vi "OxITC503 _Config_ Write AUTO-PID table.vi"(3 "error in":errorcluster, 4 "AUTOPID Table in":T1(array[cluster]), 5 "VISA session in":refnum<visa-resource-name>) -> (0 "error out":errorcluster, 1 "AUTOPID Table out":T1(array[cluster]), 2 "VISA session out":refnum<visa-resource-name>)   [LabVIEW 2013]
doc: "NOTE: this VI uses ITC503'specialist commands.\n\nWrites ITC503's AUTO-PID table. The AUTO-PID table is a 32x4 matrix of real numbers. Changes are not permanently stored (use ITC store routine to save PID table within ITC)."
panel:
  in  "Write PID Table to Instrument":bool
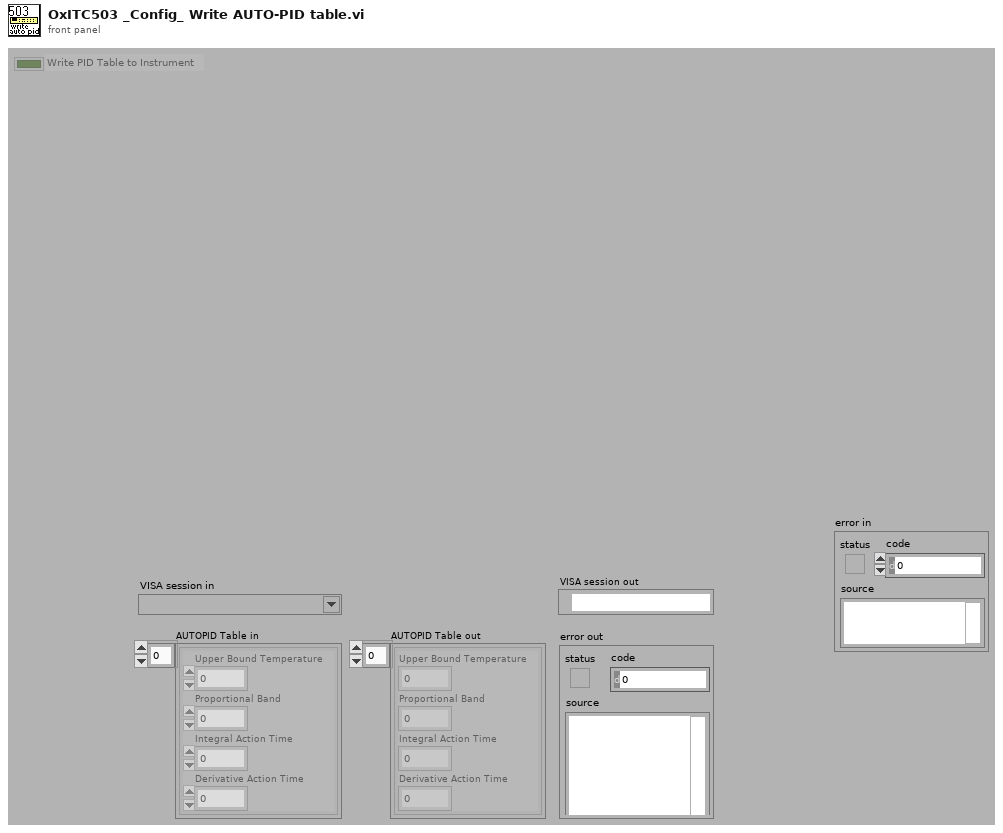
[diagram p1: front panel]
types:
  T1 = cluster{"Upper Bound Temperature":dbl, "Proportional Band":dbl, "Integral Action Time":dbl, "Derivative Action Time":dbl}[]
  T2 = cluster{"Upper Bound Temperature":dbl, "Proportional Band":dbl, "Integral Action Time":dbl, "Derivative Action Time":dbl}
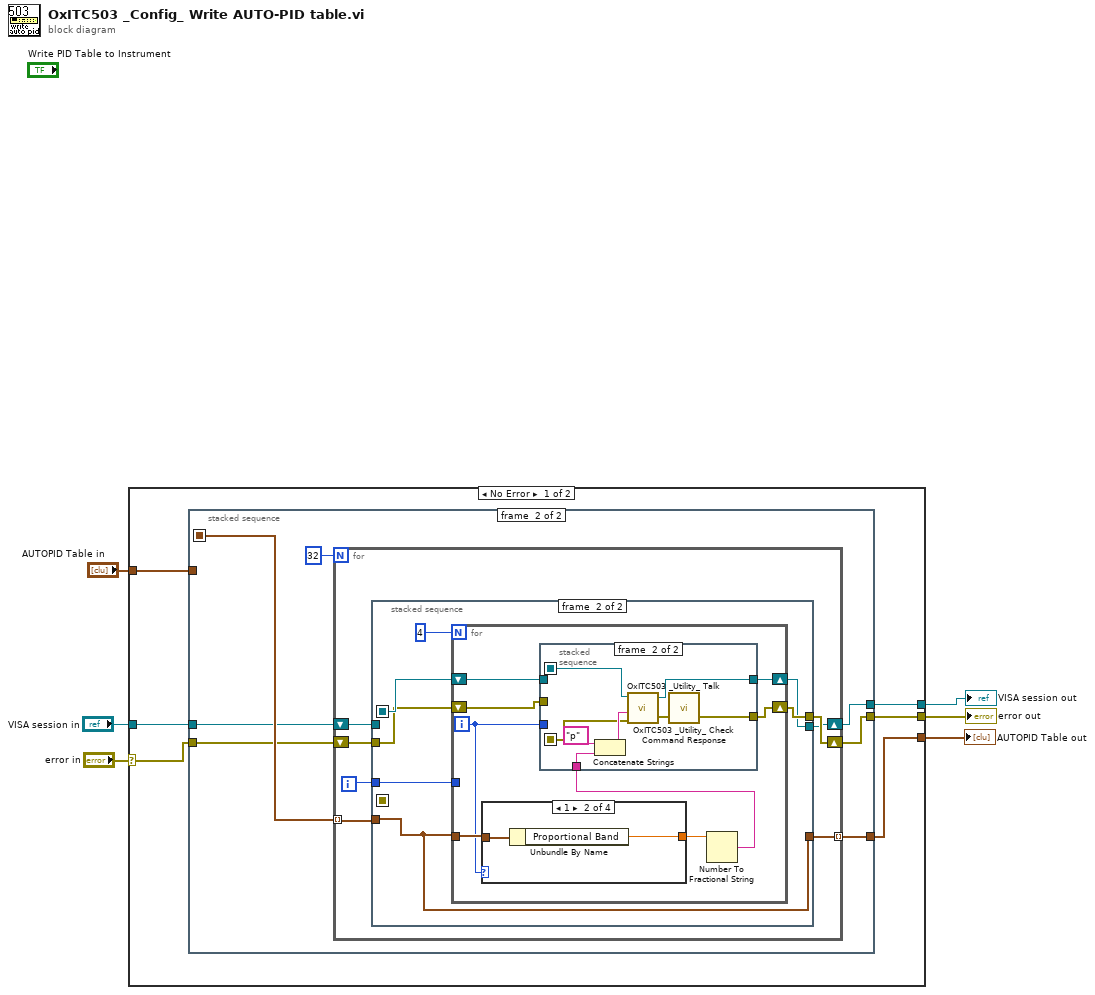
[diagram p0: block diagram]
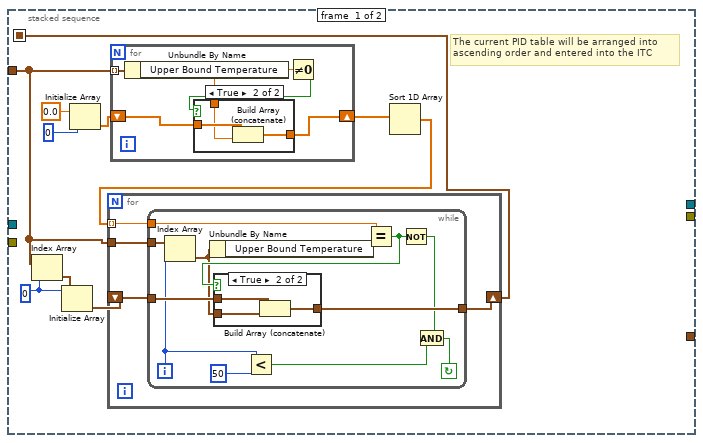
[diagram p2: hidden frame]
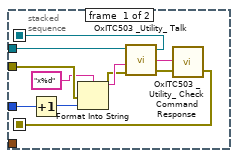
[diagram p5: hidden frame]
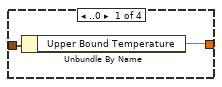
[diagram p6: hidden frame]
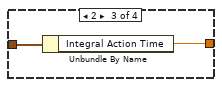
[diagram p7: hidden frame]
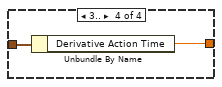
[diagram p8: hidden frame]
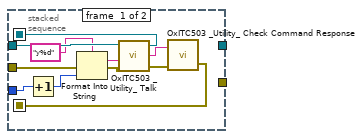
[diagram p9: hidden frame]
diagram:
  n1 = case shown="No Error" "error in" {
    selector: "error in" -> [w8 w121]
    tunnel: "AUTOPID Table in" -> [w12 w120]
    tunnel: "VISA session in" -> [w11 w119]
    tunnel: [w10 w121] -> w1
    tunnel: [w9 w120] -> w4
    tunnel: [w7 w119] -> w3
    frame No Error {
      n2 = stacked-sequence {
        seq-local: [w13 _] -> [_ w57]
        tunnel: w12 -> [w14 _]
        tunnel: w11 -> [_ w56]
        tunnel: w8 -> [_ w55]
        tunnel: [_ w54] -> w10
        tunnel: [_ w53] -> w9
        tunnel: [_ w52] -> w7
        frame #0 {
          w18 = 0
          # "The current PID table will be arranged into \nascending order and entered into the ITC"
          n3 = Index Array(array=w14, index=w18) -> (element=w17:T2)
          n4 = Initialize Array(w17, w18) -> (w15:T1)
          n5 = Initialize Array(0.0, 0) -> (w20:dbl[])
          n6 = for {
            shift-right: [w45] -> w19
            shift-left: w20 -> [w47]
            tunnel: w14 -> [w44] mode=indexing
            n7 = Unbundle By Name(w44) -> ("Upper Bound Temperature"=w43:dbl)
            n8 = Not Equal To 0?(x=w43) -> (x != 0?=w46:bool)
            n9 = case shown="True" w46 {
              tunnel: w47 -> [w48 w51]
              tunnel: [w48 w50] -> w45
              tunnel: w43 -> [_ w49]
              frame False {
              }
              frame True {
                n10 = Build Array (concatenate)(w51, w49) -> (w50:dbl[])
              }
            }
          }
          n11 = Sort 1D Array(array=w19) -> (sorted array=w16:dbl[])
          n12 = for {
            tunnel: w16 -> [w26] mode=indexing
            shift-right: [w23] -> w13
            shift-left: w15 -> [w25]
            tunnel: w14 -> [w24]
            n13 = while {
              tunnel: [w36] -> w23
              tunnel: w24 -> [w29]
              tunnel: w26 -> [w37]
              tunnel: w25 -> [w38]
              i -> [w33]
              stop <- w30 continue-if-true
              n14 = Index Array(array=w29, index=w33) -> (element=w28:T2)
              n15 = Unbundle By Name(w28) -> ("Upper Bound Temperature"=w27:dbl)
              n16 = Less?(x=w33, y=50) -> (x < y?=w31:bool)
              n17 = Equal?(x=w37, y=w27) -> (x = y?=w35:bool)
              n18 = case shown="True" w35 {
                tunnel: w38 -> [w39 w42]
                tunnel: w28 -> [_ w41]
                tunnel: [w39 w40] -> w36
                frame False {
                }
                frame True {
                  n19 = Build Array (concatenate)(w42, w41) -> (w40:T1)
                }
              }
              n20 = Not(x=w35) -> (.not. x?=w34:bool)
              n21 = And(x=w34, y=w31) -> (x .and. y?=w30:bool)
            }
          }
        }
        frame #1 {
          n22 = for {
            N: 32 -> [_]
            tunnel: w57 -> [w64] mode=indexing
            shift-right: [w61] -> w54
            shift-left: w55 -> [w62]
            shift-right: [w60] -> w52
            shift-left: w56 -> [w63]
            tunnel: [w59] -> w53 mode=indexing
            i -> [w65]
            n23 = stacked-sequence {
              seq-local: [w68 _] -> [_ w81]
              seq-local: [w67 _] -> [_ _]
              tunnel: w65 -> [w76 w82]
              tunnel: w64 -> [_ w77]
              tunnel: w63 -> [w70 _]
              tunnel: w62 -> [w69 w80]
              tunnel: [_ w79] -> w61
              tunnel: [_ w78] -> w60
              tunnel: [_ w77] -> w59
              frame #0 {
                n24 = Increment(x=w76) -> (x+1=w71:i32)
                n25 = Format Into String(format string="x%d", error in=w69, w71) -> (resulting string=w75:string, error out=w72:errorcluster)  [unwired: 1 in]
                n26 = call "OxITC503 _Utility_ Talk.vi"("VISA session"=w70, "Command"=w75, "error in (no error)"=w72) -> ("VISA session"=w68:refnum<visa-resource-name>, "read buffer"=w74:string, "error out (no error)"=w73:errorcluster)  [unwired: 2 in]
                n27 = call "OxITC503 _Utility_ Check Command Response.vi"("error in"=w73, "read buffer"=w74) -> ("error out (no error)"=w67:errorcluster)  [unwired: 1 out]
              }
              frame #1 {
                n28 = for {
                  N: 4 -> [_]
                  tunnel: w82 -> [_]
                  tunnel: w77 -> [w90]
                  shift-right: [w85] -> w79
                  shift-left: w80 -> [w86]
                  shift-right: [w84] -> w78
                  shift-left: w81 -> [w87]
                  i -> [w89]
                  n29 = case shown="1" w89 {
                    tunnel: w90 -> [w92 w94 w96 w98]
                    tunnel: [w93 w95 w97 w99] -> w88
                    frame ..0 {
                      n30 = Unbundle By Name(w92) -> ("Upper Bound Temperature"=w93:dbl)
                    }
                    frame 1 {
                      n31 = Unbundle By Name(w94) -> ("Proportional Band"=w95:dbl)
                    }
                    frame 2 {
                      n32 = Unbundle By Name(w96) -> ("Integral Action Time"=w97:dbl)
                    }
                    frame 3.. {
                      n33 = Unbundle By Name(w98) -> ("Derivative Action Time"=w99:dbl)
                    }
                  }
                  n34 = Number To Fractional String(number=w88) -> (F-format string=w91:string)  [unwired: 3 in]
                  n35 = stacked-sequence {
                    seq-local: [w102 _] -> [_ w115]
                    seq-local: [w101 _] -> [_ w114]
                    tunnel: w89 -> [w103 _]
                    tunnel: w91 -> [_ w117]
                    tunnel: w87 -> [w105 _]
                    tunnel: w86 -> [w104 _]
                    tunnel: [_ w112] -> w85
                    tunnel: [_ w111] -> w84
                    frame #0 {
                      n36 = Increment(x=w103) -> (x+1=w107:i32)
                      n37 = Format Into String(format string="y%d" ("Format String"), error in=w104, w107) -> (resulting string=w108:string, error out=w109:errorcluster)  [unwired: 1 in]
                      n38 = call "OxITC503 _Utility_ Talk.vi"("VISA session"=w105, "Command"=w108, "error in (no error)"=w109) -> ("VISA session"=w102:refnum<visa-resource-name>, "read buffer"=w110:string, "error out (no error)"=w106:errorcluster)  [unwired: 2 in]
                      n39 = call "OxITC503 _Utility_ Check Command Response.vi"("error in"=w106, "read buffer"=w110) -> ("error out (no error)"=w101:errorcluster)  [unwired: 1 out]
                    }
                    frame #1 {
                      n40 = Concatenate Strings("p", w117) -> (w116:string)
                      n41 = call "OxITC503 _Utility_ Talk.vi"("VISA session"=w115, "Command"=w116, "error in (no error)"=w114) -> ("VISA session"=w111:refnum<visa-resource-name>, "error out (no error)"=w113:errorcluster)  [unwired: 2 in, 1 out]
                      n42 = call "OxITC503 _Utility_ Check Command Response.vi"("error in"=w113) -> ("error out (no error)"=w112:errorcluster)  [unwired: 1 in, 1 out]
                    }
                  }
                }
              }
            }
          }
        }
      }
    }
    frame Error {
    }
  }
  "AUTOPID Table out" <- w4
  "VISA session out" <- w3
  "error out" <- w1
